vi "_TangoWriteDoubleImageAttribute.vi"(1 "error in":errorcluster, 2 "value":dbl[][](array[numeric]), 3 "attribute name":string, 4 "device name":string) -> (0 "error out":errorcluster)   [LabVIEW 2014, in "tango.lvlib"]
uses:
  tango.lvlib
  Insertors/base/fromDoubleImage.vi
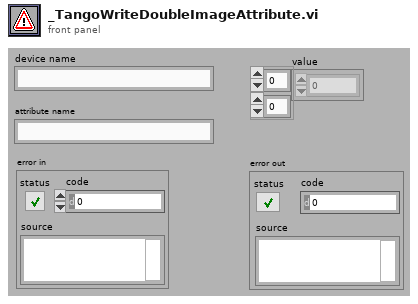
[diagram p1: front panel]
types:
  T1 = cluster{"device name":string, "attribute name":string, "quality value":i16, "quality string":string, "timestamp":dbl, "dim. x":i32, "dim. y":i32, "value":u8[], "error code":i32, "error stack":string[], "data type":u16}
  T2 = cluster{"device name":string, "attribute name":string, "quality value":i16, "quality string":string, "timestamp":dbl, "dim. x":i32, "dim. y":i32, "value":u8[], "error code":i32, "error stack":string[], "data type":u16}[]
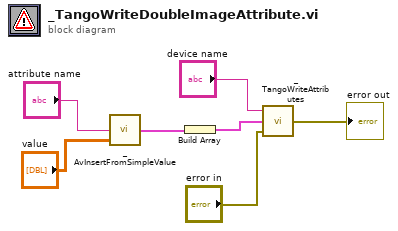
[diagram p0: block diagram]
diagram:
  n1 = call-poly "_AvInsertFromSimpleValue.vi"("value"="value", "attribute name"="attribute name") -> ("attribute value"=w4:T1)  [unwired: 1 in]
  n2 = Build Array(w4) -> (w6:T2)
  n3 = call "_TangoWriteAttributes.vi"("error in"="error in", "attribute Values"=w6, "device name"="device name") -> ("error out"=→"error out":errorcluster)
